vi "Numerric Operations.vi"() -> ()   [LabVIEW 2020]
panel:
  out "scalepwr 2":dbl
  out "Rd- Abs":dbl
  out "CmpdXOR":dbl
  out "Cmpd OR":dbl
  out "Sign Opr":dbl
  out "Rd+infinit":dbl
  out "Rd-infinity":dbl
  out "NegateD2":dbl
  out "Diff 2 (D2)":dbl
  out "Reci Pdt":dbl
  out "Sq Diff":dbl
  out "Rd off":dbl
  out "Sqrt Sum":dbl
  out "Dec Num1":dbl
  out "Inc Num2":dbl
  out "Qnt 2":dbl
  out "Rem":dbl
  out "Qnt":dbl
  out "Pdt":dbl
  out "Diff":dbl
  out "Sum":dbl
  in  "Num 2":dbl
  in  "Num 1":dbl
  # "Simple Numeric Operations"
  # "Diff 2 = Sq Diff - Reci Pdt"
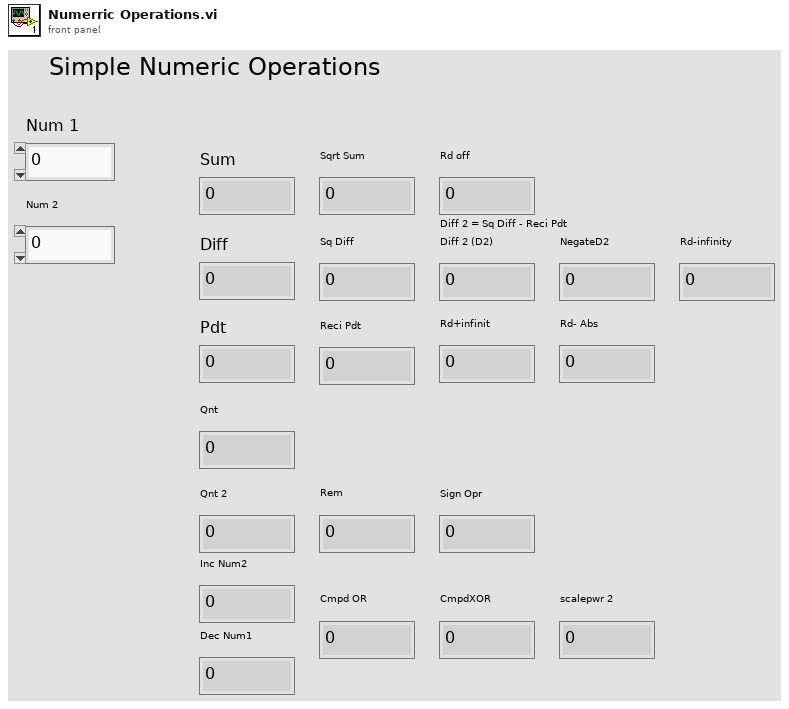
[diagram p1: front panel]
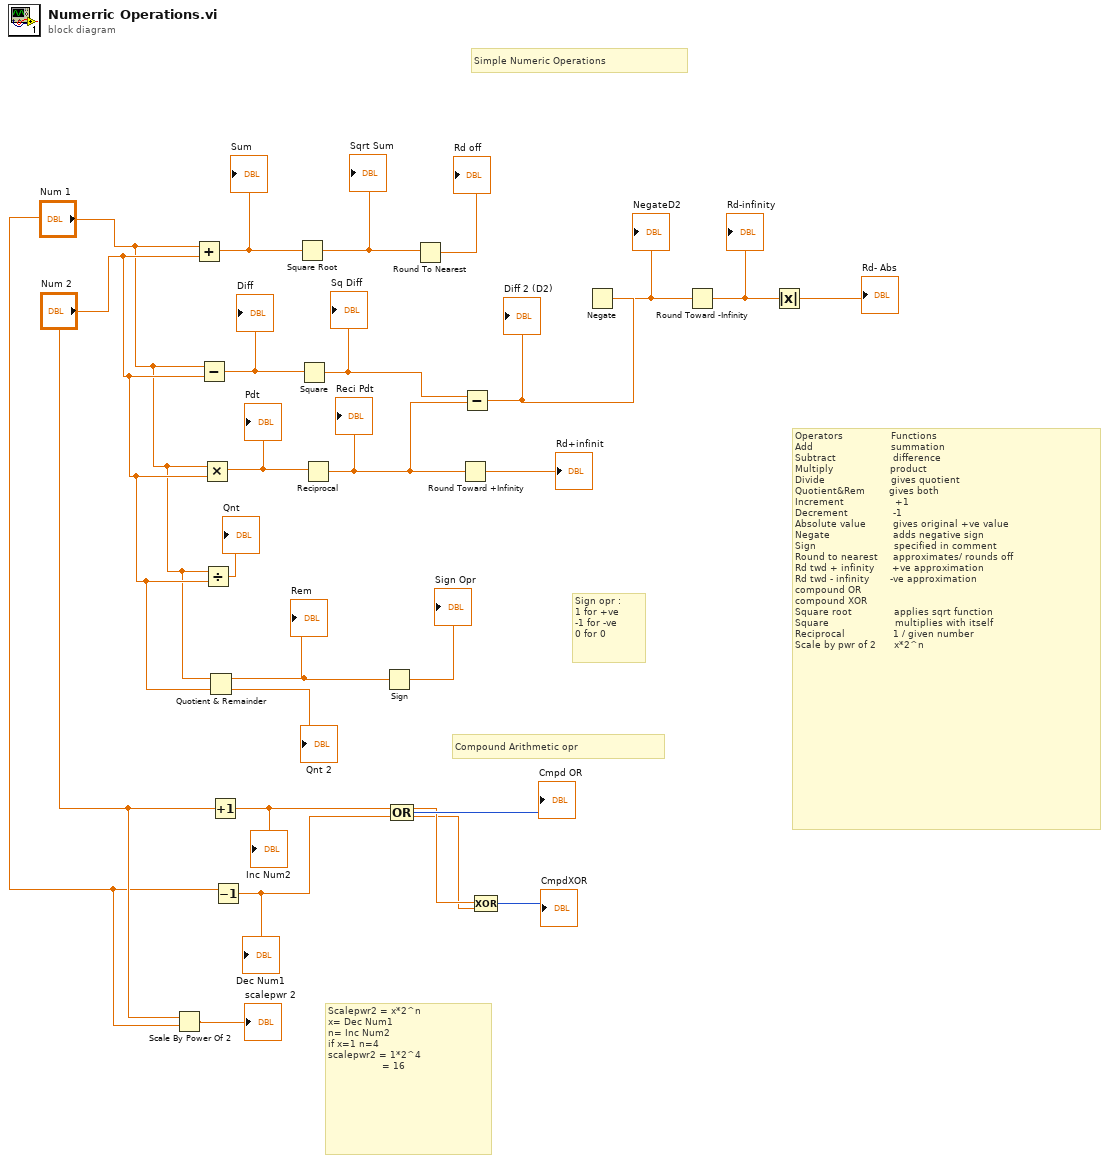
[diagram p0: block diagram]
diagram:
  # "Scalepwr2 = x*2^n\nx= Dec Num1\nn= Inc Num2\nif x=1 n=4\nscalepwr2 = 1*2^4\n                  = 16"
  # "Operators                Functions\nAdd                          summation\nSubtract                   difference\nMultiply                   product\nDivide                      gives quotient \nQuotient&Rem        gives both\nIncrement                 +1\nDecrement               -1\nAbsolute value         gives original +ve value\nNegate                     adds negative sign \nSign                          specified in comment\nRound to nearest     approximates/ rounds off\nRd twd + infinity      +ve approximation\nRd twd - infinity       -ve approximation\ncompound OR\ncompound XOR\nSquare root              applies sqrt function\nSquare                      multiplies with itself \nReciprocal                1 / given number\nScale by pwr of 2      x*2^n"
  # "Simple Numeric Operations"
  # "Sign opr :\n1 for +ve \n-1 for -ve\n0 for 0"
  # "Compound Arithmetic opr"
  n1 = Scale By Power Of 2(n="Num 2", x="Num 1") -> (x*2^n=→"scalepwr 2":dbl)
  n2 = Add(x="Num 1", y="Num 2") -> (x+y=w16:dbl)
  "Sum" <- w16
  n3 = Subtract(x="Num 1", y="Num 2") -> (x-y=w13:dbl)
  "Diff" <- w13
  n4 = Multiply(x="Num 1", y="Num 2") -> (x*y=w12:dbl)
  "Pdt" <- w12
  n5 = Divide(x="Num 1", y="Num 2") -> (x/y=→"Qnt":dbl)
  n6 = Quotient & Remainder(x="Num 1", y="Num 2") -> (x-y*floor(x/y)=w8:dbl, floor(x/y)=→"Qnt 2":dbl)
  "Rem" <- w8
  n7 = Increment(x="Num 2") -> (x+1=w19:dbl)
  "Inc Num2" <- w19
  n8 = Decrement(x="Num 1") -> (x-1=w18:dbl)
  "Dec Num1" <- w18
  n9 = Square Root(x=w16) -> (sqrt(x)=w15:dbl)
  "Sqrt Sum" <- w15
  n10 = Square(x=w13) -> (x^2=w11:dbl)
  "Sq Diff" <- w11
  n11 = Reciprocal(x=w12) -> (1/x=w7:dbl)
  "Reci Pdt" <- w7
  n12 = Sign(1:w8) -> (0:→"Sign Opr":dbl)
  n13 = Compound Arithmetic op=OR(w19, w18) -> (→"Cmpd OR":i32)
  n14 = Round To Nearest(number=w15) -> (nearest integer value=→"Rd off":dbl)
  n15 = Round Toward +Infinity(x=w7) -> (ceil(x): smallest int >= x=→"Rd+infinit":dbl)
  n16 = Subtract(x=w11, y=w7) -> (x-y=w10:dbl)
  "Diff 2 (D2)" <- w10
  n17 = Compound Arithmetic op=XOR(w19, w18) -> (→"CmpdXOR":i32)
  n18 = Negate(x=w10) -> (-x=w9:dbl)
  "NegateD2" <- w9
  n19 = Round Toward -Infinity(1:w9) -> (0:w4:dbl)
  "Rd-infinity" <- w4
  n20 = Absolute Value(x=w4) -> (abs(x)=→"Rd- Abs":dbl)
